vi "Compute Clock.vi"(6 "k-space signal in":u16[](array[numeric])=array[5000 elements], 8 "error in (no error)":errorcluster, 9 "Laser.lvclass":refnum<class "Laser.lvclass">, 10 "DAQ Class.lvclass":refnum<class "DAQ Class.lvclass">, 11 "Wavepond in":refnum<class "Wavepond.lvclass">) -> (0 "error out":errorcluster, 3 "Wavepond out":refnum<class "Wavepond.lvclass">)   [LabVIEW 2014, in "Wavepond.lvclass"]
uses:
  Wavepond.lvclass
  DAQ/DAQ Class.lvclass
  Laser/Laser.lvclass
  Wavepond.lvclass/Wavepond.ctl
  <vilib>/Analysis/baseanly.llb/Scale 1D.vi
  <vilib>/Analysis/polynomials.llb/nth Derivative of Polynomial (DBL).vi
  <vilib>/Analysis/polynomials.llb/Scalar Polynomial Evaluation (DBL).vi
  <vilib>/Analysis/NI_AALPro.lvlib
  <vilib>/Analysis/NI_AALBase.lvlib
panel:
  out "Frequency output 2":cluster{dbl[], dbl[]}[](graph)
  out "x*y":dbl[](array[numeric])
  out "Error Out":errorcluster
  in  "Error In":errorcluster
  out "frequency\nsteps":i32
  out "Frequency output":dbl[](graph)
  out "analytic phase":dbl[][](graph)
  out "original signal":dbl[](graph)
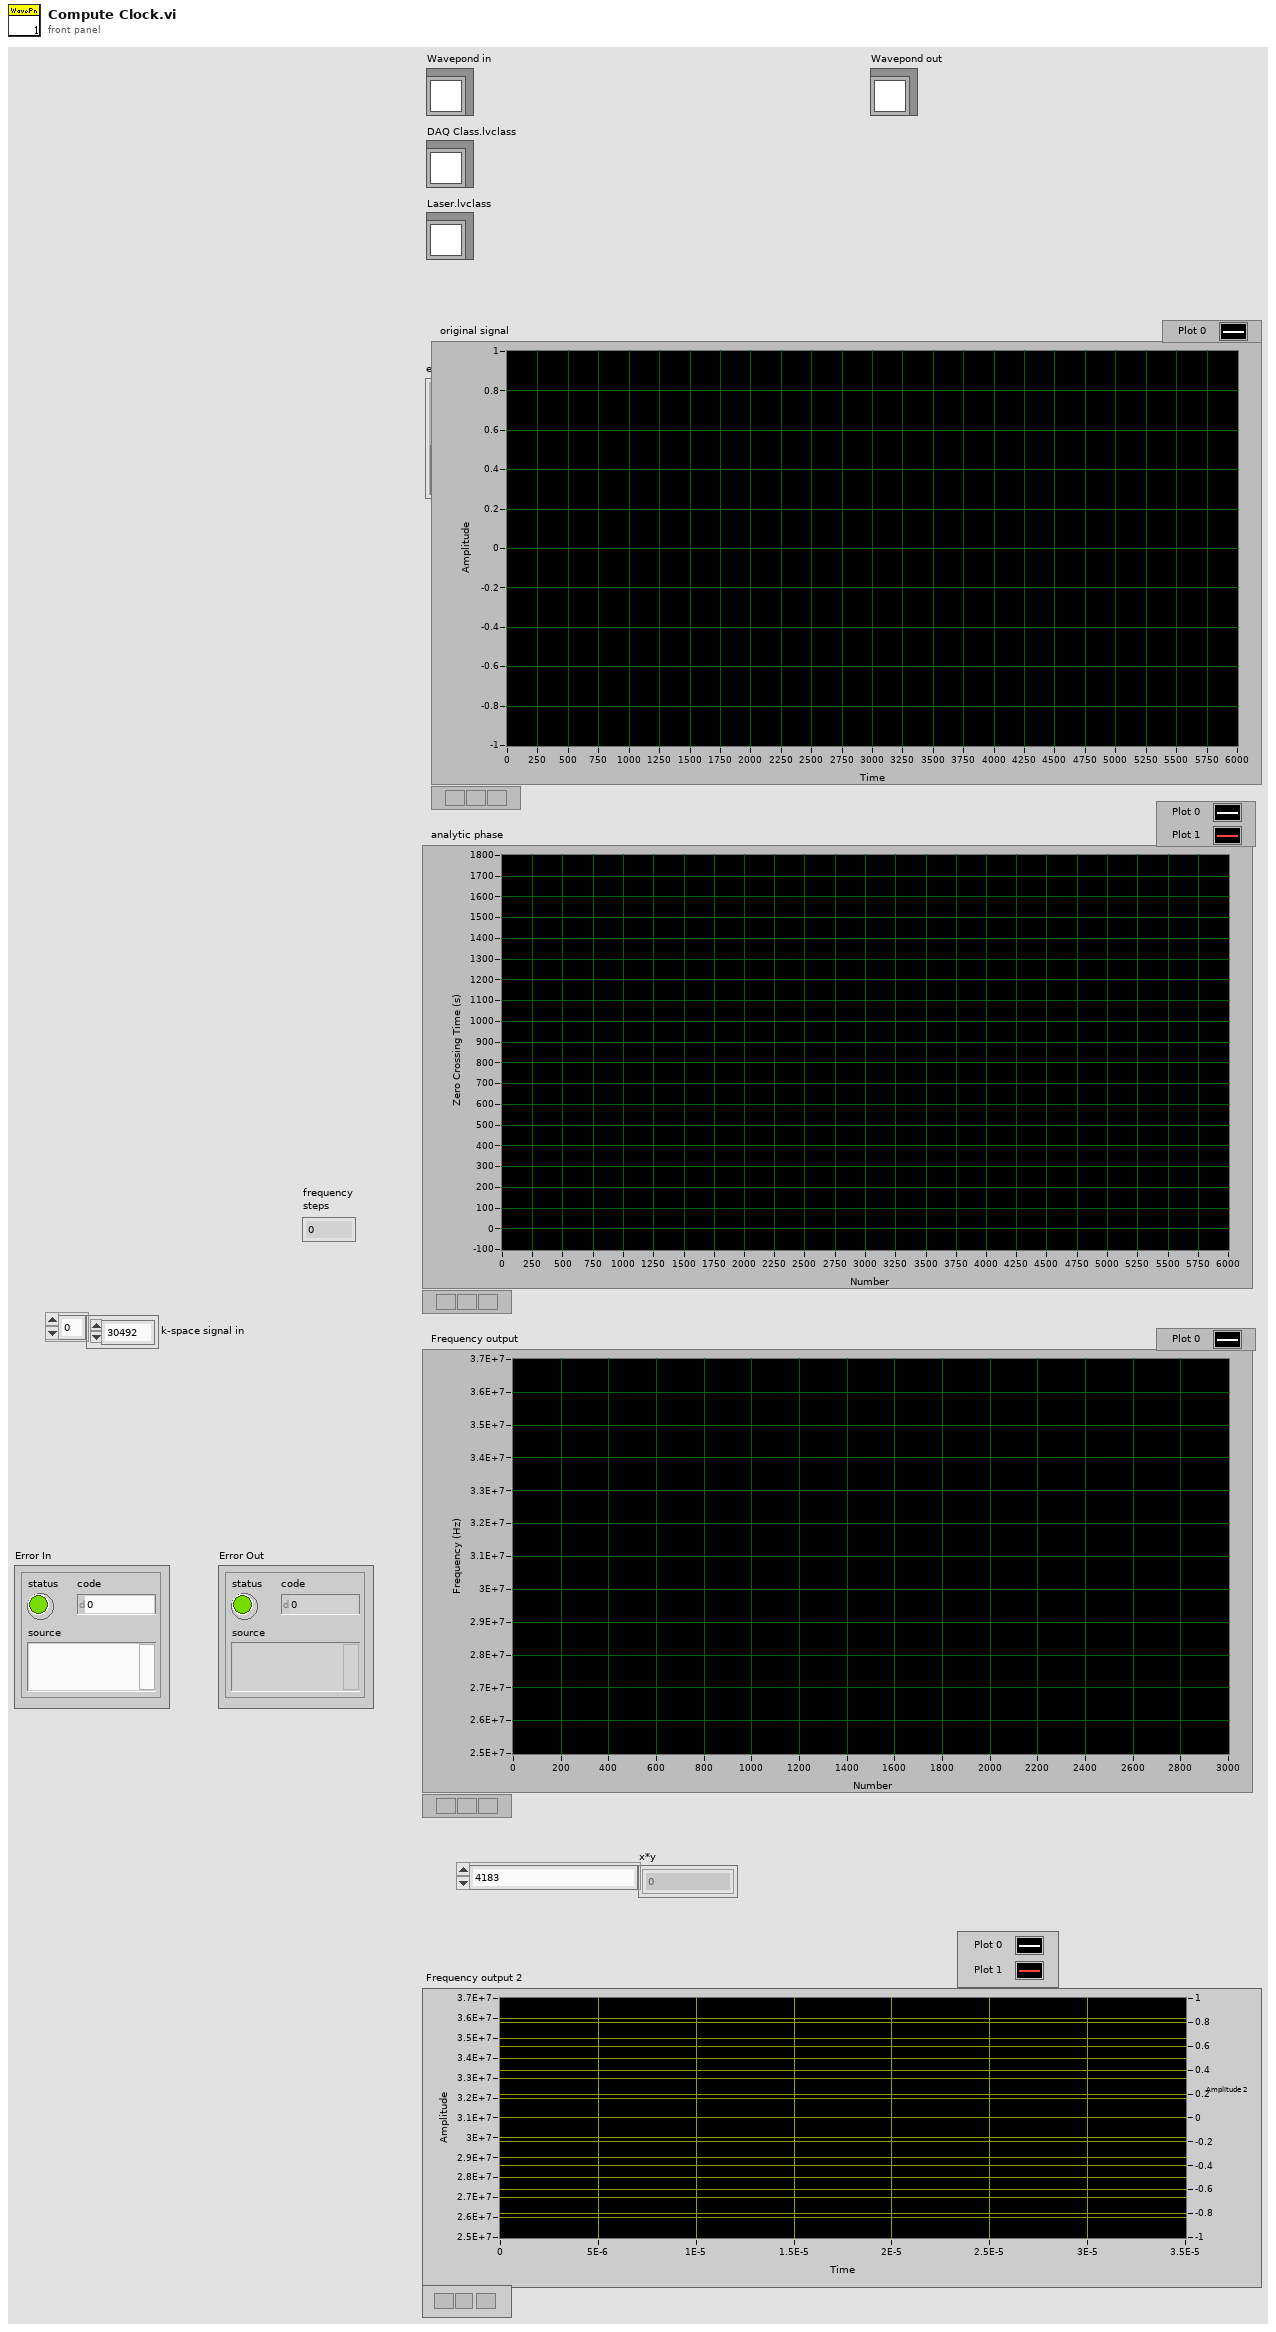
[diagram p1: front panel]
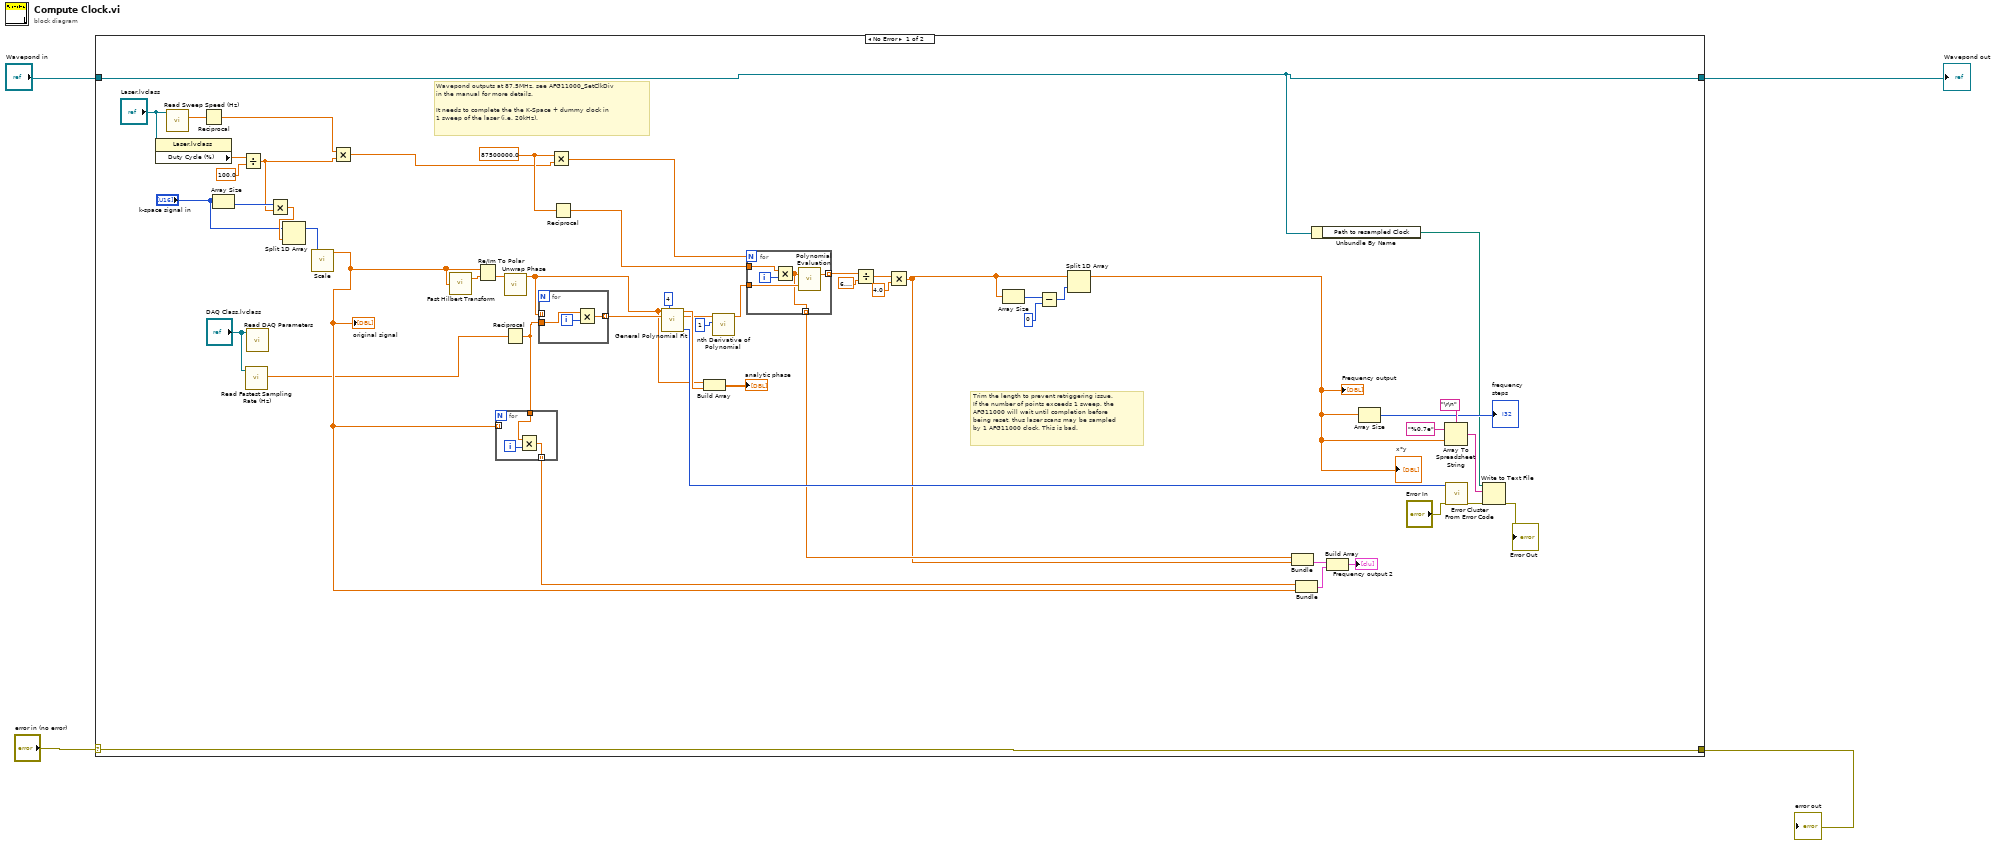
[diagram p0: block diagram]
diagram:
  n1 = case shown="No Error" "error in (no error)" {
    selector: "error in (no error)" -> [w57 w70]
    tunnel: [w57 w70] -> w3
    tunnel: [w29 w69] -> w1
    tunnel: "Wavepond in" -> [w29 w69]
    frame No Error {
      w13 = 87500000.0
      # "Trim the length to prevent retriggering issue.\nIf the number of points exceeds 1 sweep, the \nAFG11000 will wait until completion before\nbeing reset, thus laser scans may be sampled\nby 1 AFG11000 clock. This is bad."
      # "Wavepond outputs at 87.5MHz, see AFG11000_SetClkDiv\nin the manual for more details.\n\nIt needs to complete the the K-Space + dummy clock in\n1 sweep of the laser (i.e. 20kHz)."
      n2 = property class="Laser.lvclass"(reference="Laser.lvclass") -> ("Duty Cycle (%)"=w33:dbl)  [unwired: 1 in, 2 out]
      n3 = call-dynamic "Read Sweep Speed (Hz).vi"("Laser in"="Laser.lvclass") -> ("Sweep Speed (Hz)"=w28:dbl)  [unwired: 8 in, 2 out]
      n4 = Reciprocal(x=w28) -> (1/x=w6:dbl)
      n5 = Array Size(array="k-space signal in") -> (size(s)=w27:i32)
      n6 = Divide(x=w33, y=100.0) -> (x/y=w7:dbl)
      n7 = call-dynamic "Read Fastest Sampling Rate (Hz).vi"("DAQ Class in"="DAQ Class.lvclass") -> ("Fastest Sampling Rate (Hz)"=w14:dbl)  [unwired: 8 in, 2 out]
      n8 = call-dynamic "Read DAQ Parameters.vi"("DAQ Class in"="DAQ Class.lvclass") -> ()  [unwired: 8 in, 3 out]
      n9 = Multiply(x=w27, y=w7) -> (x*y=w31:dbl)
      n10 = Split 1D Array(array="k-space signal in", index=w31) -> (first subarray=w23:u16[])  [unwired: 1 out]
      n11 = call-poly <vilib>:"Scale.vi"("X"=w23) -> ("Y=(X-offset)/scale"=w17:dbl[])  [unwired: 3 out]
      "original signal" <- w17
      n12 = Multiply(x=w6, y=w7) -> (x*y=w5:dbl)
      n13 = call <vilib>:"Fast Hilbert Transform.vi"("X"=w17) -> ("Hilbert{X}"=w46:dbl[])  [unwired: 1 out]
      n14 = Re/Im To Polar(2:w46, 3:w17) -> (0:w24:dbl[])  [unwired: 1 out]
      n15 = call <vilib>:"Unwrap Phase.vi"("Phase"=w24) -> ("Unwrapped Phase"=w25:dbl[])  [unwired: 9 in, 1 out]
      n16 = Reciprocal(x=w14) -> (1/x=w20:dbl)
      n17 = for {
        tunnel: w17 -> [_] mode=indexing
        tunnel: w20 -> [w60]
        tunnel: [w58] -> w41 mode=indexing
        i -> [w59]
        n18 = Multiply(x=w60, y=w59) -> (x*y=w58:dbl)
      }
      n19 = for {
        tunnel: w25 -> [_] mode=indexing
        tunnel: [w62] -> w40 mode=indexing
        tunnel: w20 -> [w61]
        i -> [w63]
        n20 = Multiply(x=w61, y=w63) -> (x*y=w62:dbl)
      }
      n21 = Multiply(x=w13, y=w5) -> (x*y=w19:dbl)
      n22 = Reciprocal(x=w13) -> (1/x=w18:dbl)
      n23 = call <vilib>:"General Polynomial Fit.vi"("Y"=w25, "polynomial order"=4, "X"=w40) -> ("Best Polynomial Fit"=w51:dbl[], "Polynomial Coefficients"=w16:dbl[], "error"=w50:i32)  [unwired: 9 in, 1 out]
      n24 = Build Array(w25, w51) -> (→"analytic phase":dbl[][])
      n25 = call-poly <vilib>:"nth Derivative of Polynomial.vi"("order"=1, "P(x)"=w16) -> ("Nth Derivative of P(x)"=w15:dbl[])  [unwired: 8 in, 1 out]
      n26 = for {
        N: w19 -> [_]
        tunnel: w15 -> [w67]
        tunnel: [w66] -> w36 mode=indexing
        tunnel: [w65] -> w37 mode=indexing
        tunnel: w18 -> [w64]
        i -> [w68]
        n27 = Multiply(x=w64, y=w68) -> (x*y=w65:dbl)
        n28 = call-poly <vilib>:"Polynomial Evaluation.vi"("P(x)"=w67, "a"=w65) -> ("P(a)"=w66:dbl)  [unwired: 1 out]
      }
      n29 = Divide(x=w36, y=6.283185307179586) -> (x/y=w45:dbl[])
      n30 = Multiply(x=w45, y=4.0 ("P(a)")) -> (x*y=w10:dbl[])
      n31 = Array Size(array=w10) -> (size(s)=w11:i32)
      n32 = Subtract(x=w11, y=0) -> (x-y=w12:i32)
      n33 = Split 1D Array(array=w10, index=w12) -> (first subarray=w8:dbl[])  [unwired: 1 out]
      "Frequency output" <- w8
      "x*y" <- w8
      n34 = Bundle(w37, w10) -> (w38:cluster{dbl[], dbl[]})  [unwired: 1 in]
      n35 = Bundle(w41, "Y=(X-offset)/scale"=w17) -> (w42:cluster{dbl[], "Y=(X-offset)/scale":dbl[]})  [unwired: 1 in]
      n36 = Unbundle By Name(w29) -> ("Path to resampled Clock"=w30:path)
      n37 = Build Array(w38, w42) -> (→"Frequency output 2":cluster{dbl[], "Y=(X-offset)/scale":dbl[]}[])
      n38 = Array Size(array=w8) -> (size(s)=→"frequency\nsteps":i32)
      n39 = Array To Spreadsheet String(delimiter (Tab)="\r\n", array=w8, 3:"%0.7e") -> (spreadsheet string=w56:string)
      n40 = call <vilib>:"Error Cluster From Error Code.vi"("error in (no error)"="Error In", "error code (0)"=w50) -> ("error out"=w48:errorcluster)  [unwired: 7 in]
      n41 = Write to Text File(file (use dialog)=w30, text=w56, error in=w48) -> (error out=→"Error Out":errorcluster)  [unwired: 1 in, 2 out]
    }
    frame Error {
    }
  }
  "error out" <- w3
  "Wavepond out" <- w1
